vi "Archery_HS.vi"() -> ()   [LabVIEW 2014]
uses:
  <vilib>/Utility/file.llb/Write To Spreadsheet File (string).vi
  <vilib>/Utility/file.llb/Read From Spreadsheet File (string).vi
panel:
  out "Updated":bool
  in  "OK":bool
  in  "Clear":bool
  out "Highscore Table":string[][](table)
  # "Highscore"
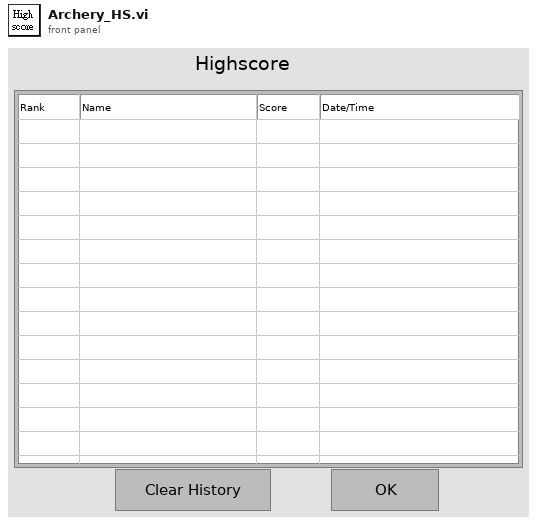
[diagram p1: front panel]
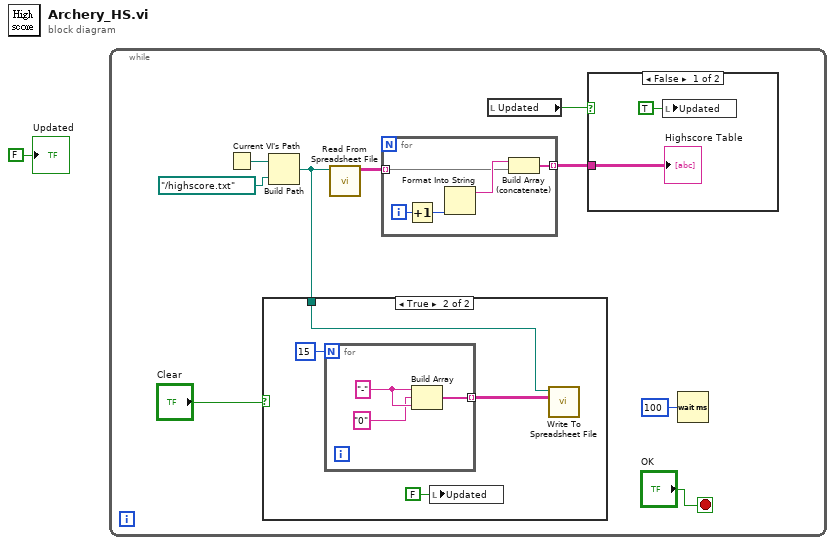
[diagram p0: block diagram]
diagram:
  n1 = while {
    stop <- "OK" stop-if-true
    n2 = Current VI's Path() -> (path=w10:path)
    n3 = Build Path(base path=w10, name or relative path=path "../highscore.txt") -> (appended path=w5:path)
    n4 = case shown="True" "Clear" {
      tunnel: w5 -> [_ w15]
      frame False {
      }
      frame True {
        n5 = for {
          N: 15 -> [_]
          tunnel: [w17] -> w14 mode=indexing
          w19 = "-"
          n6 = Build Array(w19, "0", w19) -> (w17:string[])
        }
        n7 = local write "Updated"(FALSE ("Updated")) -> ()
        n8 = call-poly <vilib>:"Write To Spreadsheet File.vi"("2D data"=w14, "file path (dialog if empty)"=w15) -> ()  [unwired: 6 in, 1 out]
      }
    }
    n9 = call-poly <vilib>:"Read From Spreadsheet File.vi"("file path (dialog if empty)"=w5) -> ("all rows"=w8:string[][])  [unwired: 6 in, 4 out]
    n10 = for {
      tunnel: w8 -> [w21] mode=indexing
      tunnel: [w20] -> w2 mode=indexing
      i -> [w24]
      n11 = Increment(x=w24) -> (x+1=w23:i32)
      n12 = Format Into String(w23) -> (resulting string=w22:string)  [unwired: 3 in, 1 out]
      n13 = Build Array (concatenate)(w22, w21) -> (w20:string[])
    }
    n14 = local read "Updated"() -> (w3:bool)
    n15 = case shown="False" w3 {
      tunnel: w2 -> [w12 _]
      frame False {
        n16 = local write "Updated"(TRUE ("Updated")) -> ()
        "Highscore Table" <- w12
      }
      frame True {
      }
    }
    n17 = Wait (ms)(milliseconds to wait=u32 100) -> ()  [unwired: 1 out]
  }
  "Updated" <- FALSE ("Updated")
